vi "Check Multiple.vi"(6 "Offset":i32, 8 "error in (no error)":errorcluster, 10 "Divisor":i32, 11 "Mapping":u16) -> (0 "error out":errorcluster)   [LabVIEW 2020, in "Modbus Master System Explorer.lvlib"]
uses:
  Modbus Master System Explorer.lvlib
  <vilib>/ErrorRing/Error Ring.xnode
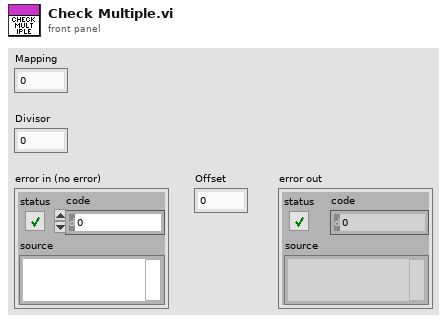
[diagram p1: front panel]
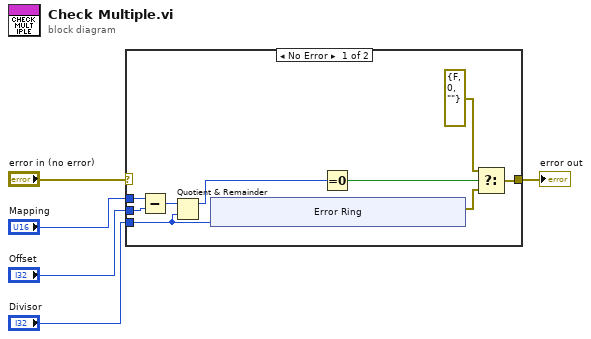
[diagram p0: block diagram]
diagram:
  n1 = case shown="No Error" "error in (no error)" {
    selector: "error in (no error)" -> [_ w20]
    tunnel: "Divisor" -> [w11 _]
    tunnel: "Mapping" -> [w8 _]
    tunnel: [w12 w20] -> w2
    tunnel: "Offset" -> [w7 _]
    frame No Error {
      n2 = Subtract(x=w8, y=w7) -> (x-y=w6:i32)
      n3 = Quotient & Remainder(x=w6, y=w11) -> (x-y*floor(x/y)=w14:i32)  [unwired: 1 out]
      n4 = xnode "Error Ring"("parameter 0"=w11) -> ("error out"=w10:errorcluster)
      n5 = Equal To 0?(x=w14) -> (x = 0?=w13:bool)
      n6 = Select(t=errorcluster {"status"=FALSE, "code"=0, "source"=""} ("f"), s=w13, f=w10) -> (s? t:f=w12:errorcluster)
    }
    frame Error {
    }
  }
  "error out" <- w2
